vi "Set Target Groups (Name Map).vi"(8 "error in (no error)":errorcluster, 10 "Target Groups":map{string, T1}(c390), 11 "TCPMessaging in":refnum<class "TCPMessaging.lvclass">) -> (0 "error out":errorcluster, 3 "TCPMessaging out":refnum<class "TCPMessaging.lvclass">)   [LabVIEW 2020, in "Vecto.lvlib" / "TCPMessaging.lvclass"]
uses:
  TCPMessaging.lvclass
  TCPMessaging.lvclass/TCPMessaging.ctl
  Target Group.ctl
  Vecto.lvlib
  VectoConfig/Target Group Info.ctl
  VectoConfig/VectoConfig.lvlib
  Node Name ID.ctl
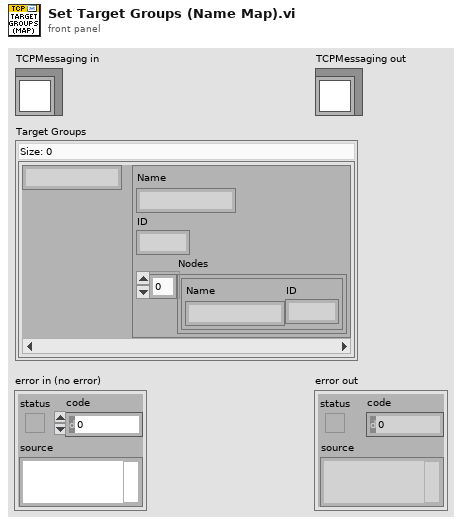
[diagram p1: front panel]
types:
  T1 = typedef "VectoConfig.lvlib/Target Group Info.ctl" = cluster{"Name":string, "ID":u32, "Nodes":T2[]}
  T2 = typedef "Vecto.lvlib/Node Name ID.ctl" = cluster{"Name":string, "ID":u32}
  T3 = typedef "Vecto.lvlib/Target Group.ctl" = cluster{"Node":u32, "Groups":u32[]}
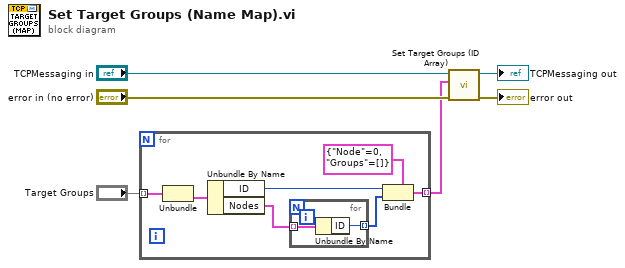
[diagram p0: block diagram]
diagram:
  n1 = for {
    tunnel: "Target Groups" -> [w13] mode=indexing
    tunnel: [w8] -> w1 mode=indexing
    n2 = Unbundle(w13) -> ("Info"=w12:T1)  [unwired: 1 out]
    n3 = Unbundle By Name(w12) -> ("ID"=w10:u32, "Nodes"=w11:T2[])
    n4 = for {
      tunnel: w11 -> [w15] mode=indexing
      tunnel: [w14] -> w9 mode=indexing
      n5 = Unbundle By Name(w15) -> ("ID"=w14:u32)
    }
    n6 = Bundle(cluster=T3 {"Node"=0, "Groups"=[]} ("Node Group"), "Node"=w10, "Groups"=w9) -> (w8:T3)
  }
  n7 = call "Set Target Groups (ID Array).vi"("error in (no error)"="error in (no error)", "Target Groups"=w1, "TCPMessaging in"="TCPMessaging in") -> ("error out"=→"error out":errorcluster, "TCPMessaging out"=→"TCPMessaging out":refnum<class "TCPMessaging.lvclass">)  [unwired: 7 in]
